vi "Set SR830 source (SubVI).vi"(9 "freq":dbl, 10 "voltage":dbl, 11 "VISA引用句柄输入":refnum<visa-resource-name>) -> ()   [LabVIEW 2019, in "User lib.lvlib"]
uses:
  User lib.lvlib
panel:
  in  "Internal Reference Frequency (1000 Hz)":dbl=1000.0
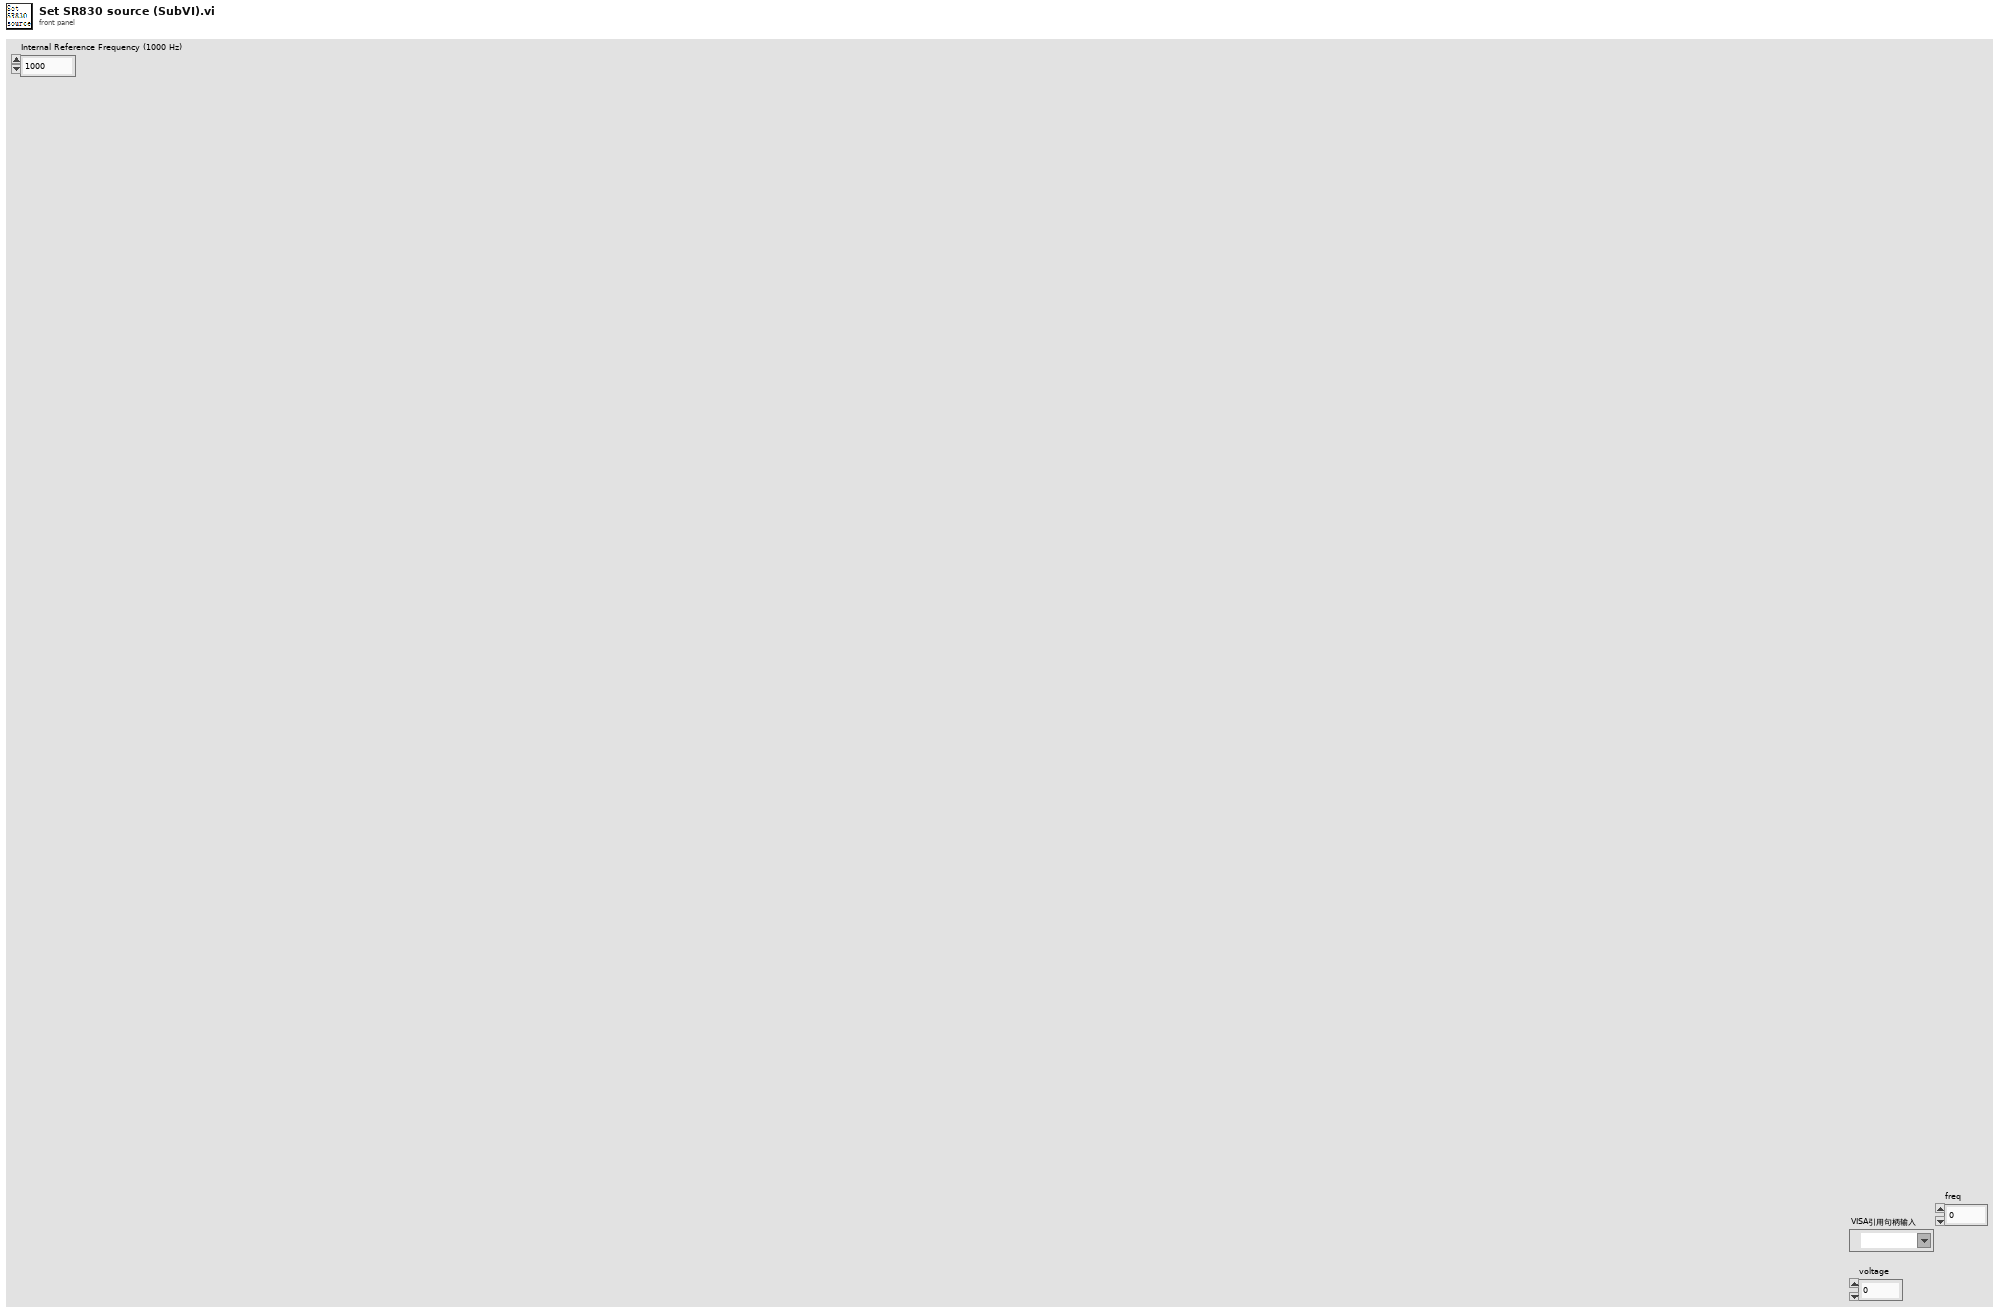
[diagram p1: front panel]
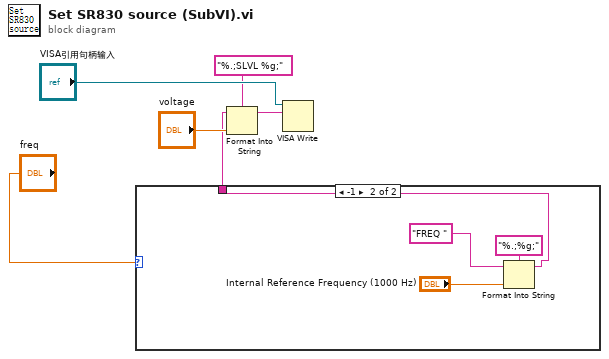
[diagram p0: block diagram]
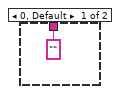
[diagram p2: hidden frame]
diagram:
  n1 = case shown="-1" "freq" {
    tunnel: ["" w8] -> w2
    frame 0, Default {
    }
    frame -1 {
      n2 = Format Into String(format string="%.;%g;", initial string="FREQ ", "Internal Reference Frequency (1000 Hz)") -> (resulting string=w8:string)  [unwired: 1 in, 1 out]
    }
  }
  n3 = Format Into String(format string="%.;SLVL %g;", initial string=w2, "voltage") -> (resulting string=w4:string)  [unwired: 1 in, 1 out]
  n4 = VISA Write(VISA resource name="VISA引用句柄输入", write buffer=w4) -> ()  [unwired: 1 in, 3 out]
